vi "Test.vi"() -> ()   [LabVIEW 2017]
uses:
  Framework/Robot Global Data.vi
panel:
  in  "Numeric":dbl
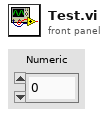
[diagram p1: front panel]
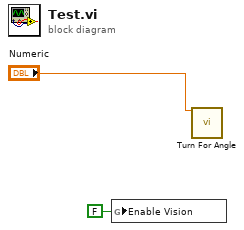
[diagram p0: block diagram]
diagram:
  n1 = global write "Robot Global Data.vi" "Enable Vision"(FALSE ("Enable Vision")) -> ()
  n2 = call "Turn For Angle.vi"("Speed"="Numeric") -> ()  [unwired: 13 in, 2 out]
